vi "Get Central Message Handler DVR.vi"(8 "Error In":errorcluster, 11 "Central Message Handler In":refnum<class "Central Message Handler.lvclass">) -> (0 "Error Out":errorcluster, 2 "DVR":refnum<data-value>, 3 "Central Message Handler Out":refnum<class "Central Message Handler.lvclass">)   [LabVIEW 2019, in "Central Message Handler.lvclass"]
uses:
  Central Message Handler.lvclass
  Controls/Data.ctl
  Public/Controls/Message.ctl
  Process/Public/Controls/Process Message.ctl
  Central Message Handler.lvclass/Central Message Handler.ctl
  Utilities/Utilities.lvlib
  Process/Process.lvclass
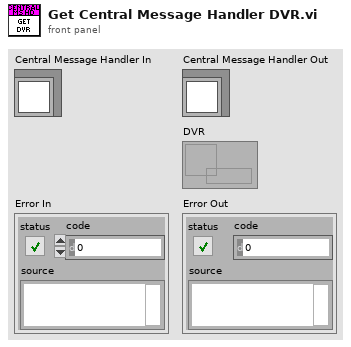
[diagram p1: front panel]
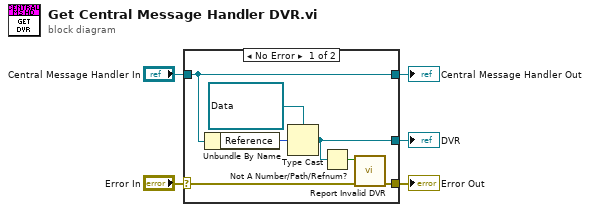
[diagram p0: block diagram]
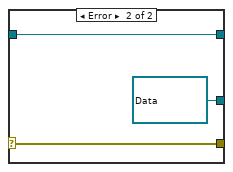
[diagram p2: hidden frame]
diagram:
  n1 = case shown="No Error" "Error In" {
    selector: "Error In" -> [w7 w15]
    tunnel: "Central Message Handler In" -> [w11 w14]
    tunnel: [w6 w15] -> w2
    tunnel: [w11 w14] -> w4
    tunnel: [w9 refnum<data-value> refnum ("data value reference")] -> w1
    frame No Error {
      n2 = Unbundle By Name(w11) -> ("Reference"=w12:u64)
      n3 = Type Cast(type=refnum<data-value> refnum ("data value reference"), x=w12) -> (*(type *) &x=w9:refnum<data-value>)
      n4 = Not A Number/Path/Refnum?(number/path/refnum=w9) -> (NaN/Path/Refnum?=w8:bool)
      n5 = call "Report Invalid DVR.vi"("Error In"=w7, "Invalid DVR"=w8) -> ("Error Out"=w6:errorcluster)  [unwired: 9 in]
    }
    frame Error {
    }
  }
  "Error Out" <- w2
  "Central Message Handler Out" <- w4
  "DVR" <- w1
